vi "run_single_technique.vi"() -> ()   [LabVIEW 2014, in "machine.lvclass"]
uses:
  machine.lvclass
  machine.lvclass/machine.ctl
panel:
  in  "input_machine_reference.lvclass":refnum<class "machine.lvclass">
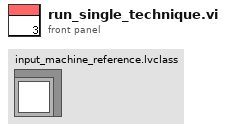
[diagram p1: front panel]
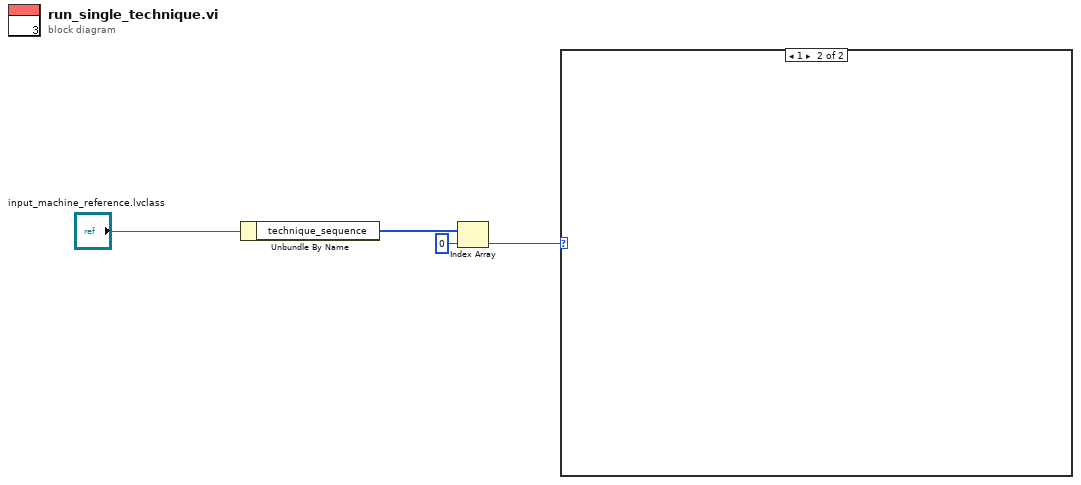
[diagram p0: block diagram]
diagram:
  n1 = Unbundle By Name("input_machine_reference.lvclass") -> ("technique_sequence"=w3:u32[])
  n2 = Index Array(array=w3, index=0) -> (element=w1:u32)
  n3 = case shown="1" w1 {
    frame 0, Default {
    }
    frame 1 {
    }
  }
